vi "Add Index (U32).vi"(7 "Count":i32, 8 "Enabled":bool, 9 "Word":u32, 10 "Indices Input":i32[](array[numeric])) -> (0 "Count+1":i32, 3 "Indices Output":i32[](array[numeric]))   [LabVIEW 2011]
uses:
  GlobalVariables.vi
panel:
  in  "Dnet Output Words":u32[](array[numeric])
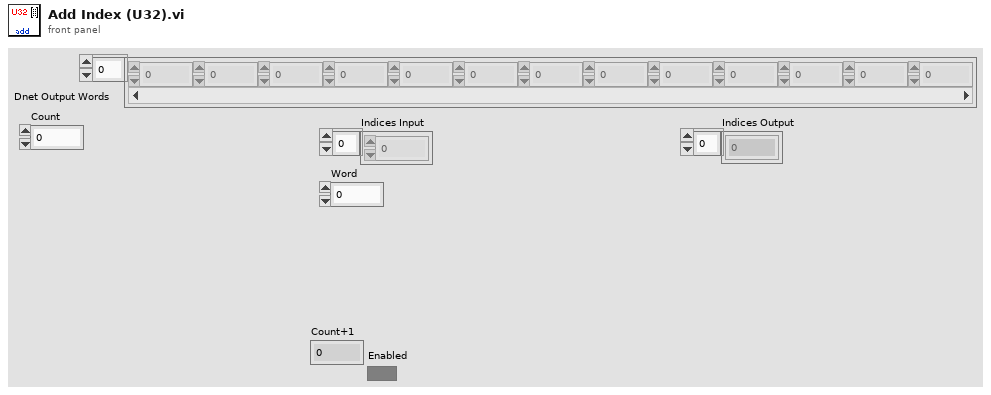
[diagram p1: front panel]
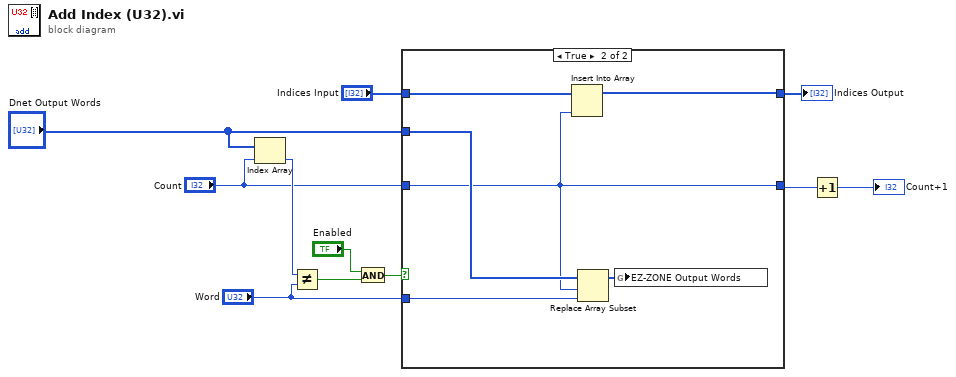
[diagram p0: block diagram]
diagram:
  n1 = Index Array(array="Dnet Output Words", index="Count") -> (element=w11:u32)
  n2 = Not Equal?(x=w11, y="Word") -> (x != y?=w6:bool)
  n3 = And(x="Enabled", y=w6) -> (x .and. y?=w5:bool)
  n4 = case shown="True" w5 {
    tunnel: "Dnet Output Words" -> [_ w18]
    tunnel: "Indices Input" -> [w13 w17]
    tunnel: [w13 w16] -> w9
    tunnel: "Word" -> [_ w15]
    tunnel: "Count" -> [w12 w14]
    tunnel: [w12 w14] -> w1
    frame False {
    }
    frame True {
      n5 = Insert Into Array(array=w17, new element=w14) -> (w16:i32[])  [unwired: 1 in]
      n6 = Replace Array Subset(array=w18, new element=w15, index=w14) -> (w19:u32[])
      n7 = global write "GlobalVariables.vi" "EZ-ZONE Output Words"(w19) -> ()
    }
  }
  "Indices Output" <- w9
  n8 = Increment(x=w1) -> (x+1=→"Count+1":i32)
